vi "LSTM-cell-2 (SubVI).vi"(7 "x":T1, 9 "h":T1, 11 "c":T1) -> (1 "h + 1":T1, 3 "c + 1":T1)   [LabVIEW 2020]
uses:
  <vilib>/Analysis/Matrix/Datatypes/RealMatrix.ctl
  <vilib>/Analysis/7linalg.llb/Real Transpose Matrix.vi
  <vilib>/Analysis/Matrix/Numeric/Conversions/Array To Matrix - RA2.vi
  <vilib>/Analysis/Matrix/Numeric/Add/Add - RM,RM.vi
  <vilib>/Analysis/Matrix/NI_Matrix.lvlib
  <vilib>/Analysis/NI_AALPro.lvlib
panel:
  out "indicator":T1
  in  "bi":T1
  in  "Ui":T1
  in  "Wi":T1
  in  "bc":T1
  in  "Uc":T1
  in  "Wc":T1
  in  "bf":T1
  in  "Uf":T1
  in  "Wf":T1
  in  "bo":T1
  in  "Uo":T1
  in  "Wo":T1
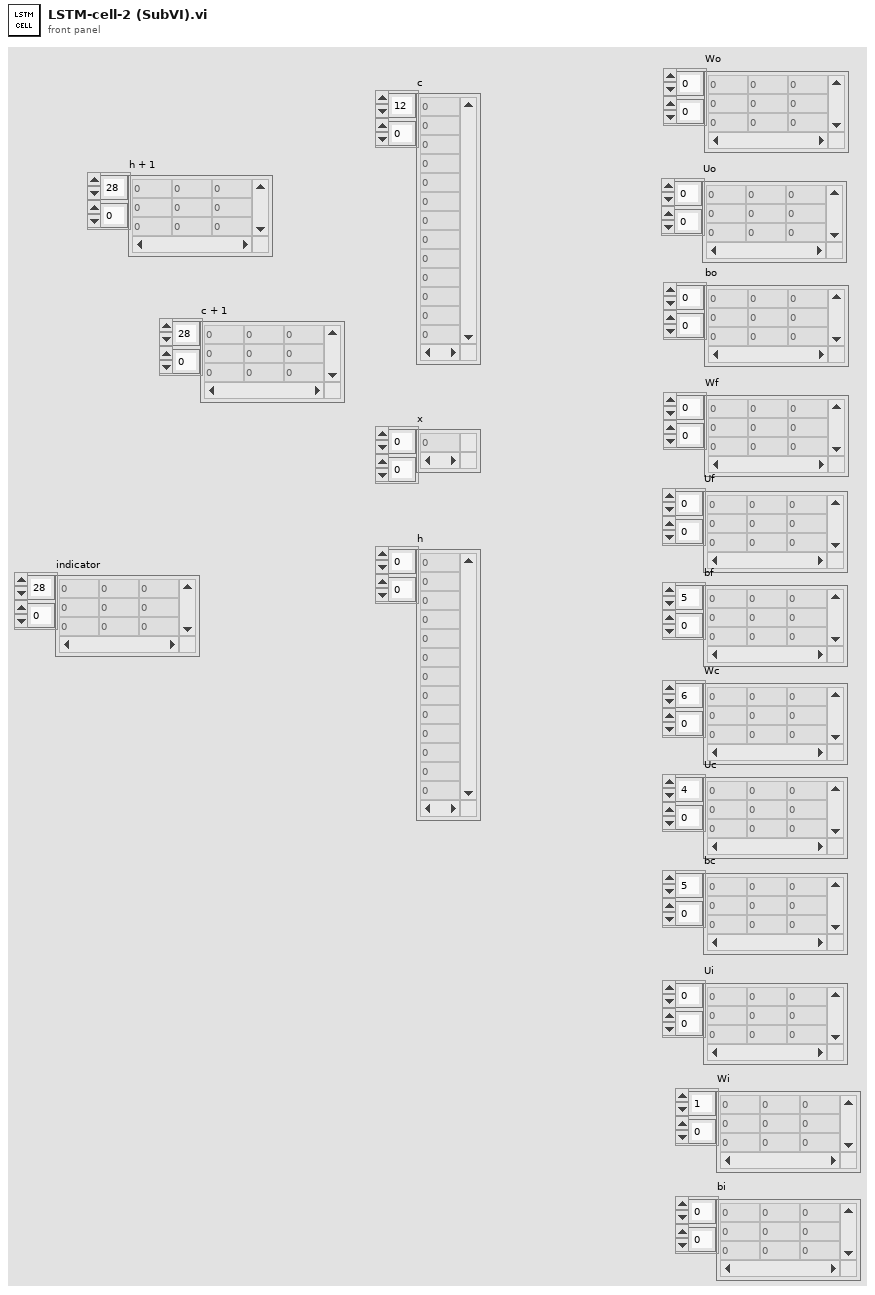
[diagram p1: front panel]
types:
  T1 = typedef "NI_Matrix.lvlib/RealMatrix.ctl" = dbl[][]
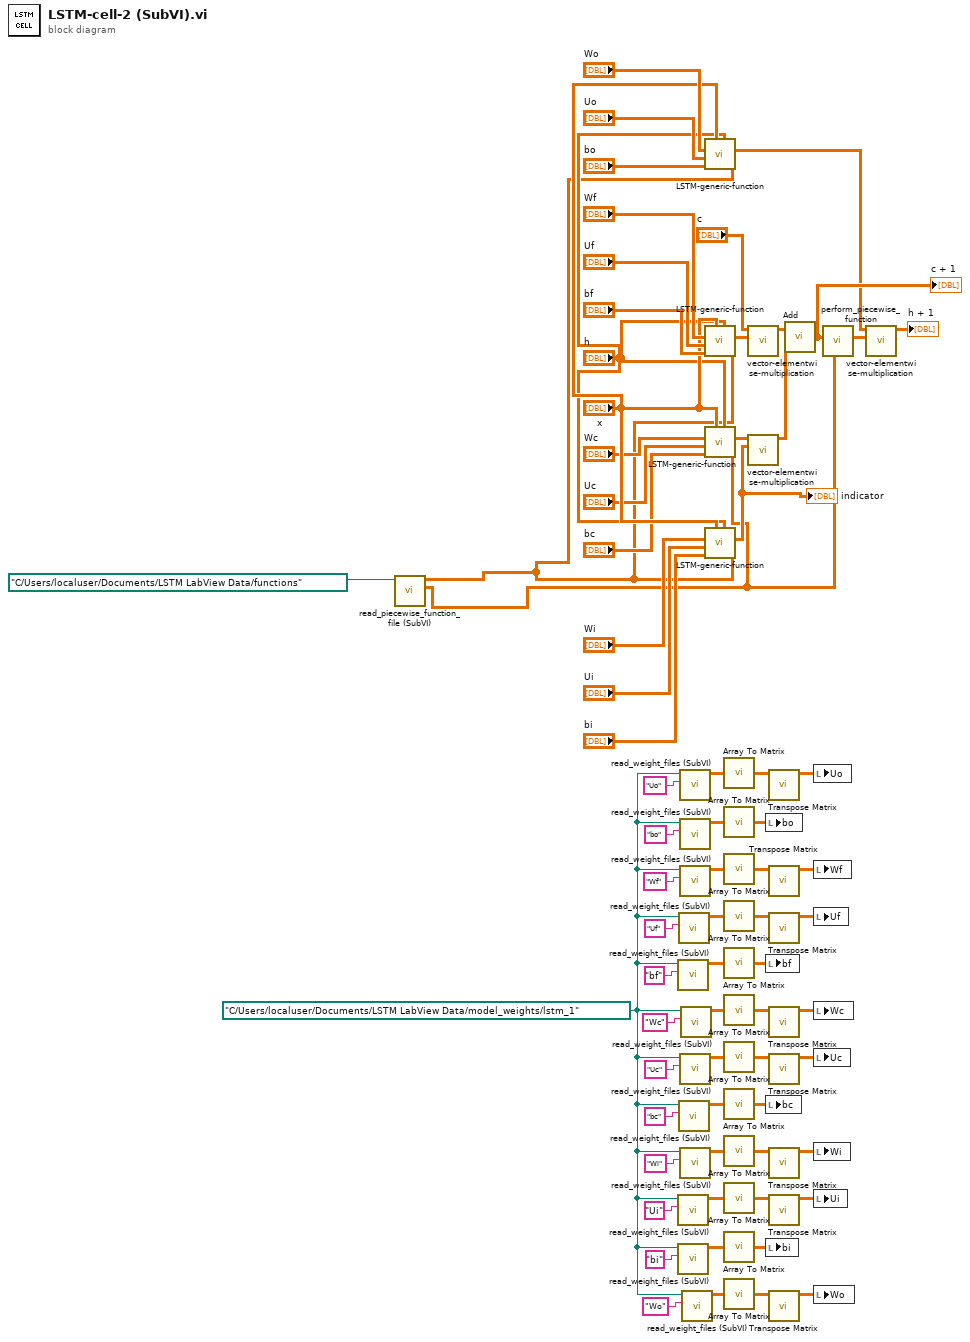
[diagram p0: block diagram]
diagram:
  w46 = path "C:/Users/localuser/Documents/LSTM LabView Data/model_weights/lstm_1" ("cell 1 path")
  n1 = call "read_piecewise_function_file (SubVI).vi"("Path"=path "C:/Users/localuser/Documents/LSTM LabView Data/functions" ("functions path")) -> ("arctan"=w1:dbl[][], "sigmoid"=w2:dbl[][])  [unwired: 9 in]
  n2 = call "read_weight_files (SubVI).vi"("weight file name"="bf" ("String"), "weights path"=w46) -> ("all rows"=w66:dbl[][])  [unwired: 9 in]
  n3 = call "read_weight_files (SubVI).vi"("weight file name"="Ui" ("String"), "weights path"=w46) -> ("all rows"=w60:dbl[][])  [unwired: 9 in]
  n4 = call "read_weight_files (SubVI).vi"("weight file name"="bi" ("String"), "weights path"=w46) -> ("all rows"=w67:dbl[][])  [unwired: 9 in]
  n5 = call "read_weight_files (SubVI).vi"("weight file name"="Uf" ("String"), "weights path"=w46) -> ("all rows"=w62:dbl[][])  [unwired: 9 in]
  n6 = call "read_weight_files (SubVI).vi"("weight file name"="bc" ("String"), "weights path"=w46) -> ("all rows"=w68:dbl[][])  [unwired: 9 in]
  n7 = call "read_weight_files (SubVI).vi"("weight file name"="Uo" ("String"), "weights path"=w46) -> ("all rows"=w65:dbl[][])  [unwired: 9 in]
  n8 = call "read_weight_files (SubVI).vi"("weight file name"="bo" ("String"), "weights path"=w46) -> ("all rows"=w64:dbl[][])  [unwired: 9 in]
  n9 = call "read_weight_files (SubVI).vi"("weight file name"="Wf" ("String"), "weights path"=w46) -> ("all rows"=w63:dbl[][])  [unwired: 9 in]
  n10 = call "read_weight_files (SubVI).vi"("weight file name"="Uc" ("String"), "weights path"=w46) -> ("all rows"=w58:dbl[][])  [unwired: 9 in]
  n11 = call "read_weight_files (SubVI).vi"("weight file name"="Wi" ("String"), "weights path"=w46) -> ("all rows"=w61:dbl[][])  [unwired: 9 in]
  n12 = call "read_weight_files (SubVI).vi"("weight file name"="Wc" ("String"), "weights path"=w46) -> ("all rows"=w59:dbl[][])  [unwired: 9 in]
  n13 = call "read_weight_files (SubVI).vi"("weight file name"="Wo" ("String"), "weights path"=w46) -> ("all rows"=w45:dbl[][])  [unwired: 9 in]
  n14 = call "LSTM-generic-function.vi"("piecewise function"=w2, "h"="h", "x"="x", "b"="bo", "U"="Uo", "W"="Wo") -> ("y"=w21:T1)  [unwired: 5 in]
  n15 = call "LSTM-generic-function.vi"("piecewise function"=w2, "h"="h", "x"="x", "b"="bf", "U"="Uf", "W"="Wf") -> ("y"=w69:T1)  [unwired: 5 in]
  n16 = call "LSTM-generic-function.vi"("piecewise function"=w1, "h"="h", "x"="x", "b"="bc", "U"="Uc", "W"="Wc") -> ("y"=w70:T1)  [unwired: 5 in]
  n17 = call "LSTM-generic-function.vi"("piecewise function"=w2, "h"="h", "x"="x", "b"="bi", "U"="Ui", "W"="Wi") -> ("y"=w4:T1)  [unwired: 5 in]
  "indicator" <- w4
  n18 = call-poly <vilib>:"Array To Matrix.vi"("Real 2D Array"=w65) -> ("Real Matrix"=w42:T1)
  n19 = call-poly <vilib>:"Array To Matrix.vi"("Real 2D Array"=w64) -> ("Real Matrix"=w31:T1)
  n20 = call-poly <vilib>:"Array To Matrix.vi"("Real 2D Array"=w63) -> ("Real Matrix"=w37:T1)
  n21 = call-poly <vilib>:"Array To Matrix.vi"("Real 2D Array"=w62) -> ("Real Matrix"=w40:T1)
  n22 = call-poly <vilib>:"Array To Matrix.vi"("Real 2D Array"=w66) -> ("Real Matrix"=w28:T1)
  n23 = call-poly <vilib>:"Array To Matrix.vi"("Real 2D Array"=w59) -> ("Real Matrix"=w38:T1)
  n24 = call-poly <vilib>:"Array To Matrix.vi"("Real 2D Array"=w58) -> ("Real Matrix"=w41:T1)
  n25 = call-poly <vilib>:"Array To Matrix.vi"("Real 2D Array"=w68) -> ("Real Matrix"=w25:T1)
  n26 = call-poly <vilib>:"Array To Matrix.vi"("Real 2D Array"=w61) -> ("Real Matrix"=w36:T1)
  n27 = call-poly <vilib>:"Array To Matrix.vi"("Real 2D Array"=w60) -> ("Real Matrix"=w39:T1)
  n28 = call-poly <vilib>:"Array To Matrix.vi"("Real 2D Array"=w67) -> ("Real Matrix"=w22:T1)
  n29 = call-poly <vilib>:"Array To Matrix.vi"("Real 2D Array"=w45) -> ("Real Matrix"=w43:T1)
  n30 = call "vector-elementwise-multiplication.vi"("Matrix in"=w69, "Matrix 1"="c") -> ("elementwise product"=w19:T1)  [unwired: 9 in]
  n31 = call "vector-elementwise-multiplication.vi"("Matrix in"=w4, "Matrix 1"=w70) -> ("elementwise product"=w71:T1)  [unwired: 9 in]
  n32 = local write "bo"(w31) -> ()
  n33 = local write "bf"(w28) -> ()
  n34 = local write "bc"(w25) -> ()
  n35 = local write "bi"(w22) -> ()
  n36 = call-poly <vilib>:"Transpose Matrix.vi"("Input Matrix"=w42) -> ("Matrix Transpose"=w32:T1)  [unwired: 9 in, 1 out]
  n37 = call-poly <vilib>:"Transpose Matrix.vi"("Input Matrix"=w37) -> ("Matrix Transpose"=w30:T1)  [unwired: 9 in, 1 out]
  n38 = call-poly <vilib>:"Transpose Matrix.vi"("Input Matrix"=w40) -> ("Matrix Transpose"=w29:T1)  [unwired: 9 in, 1 out]
  n39 = call-poly <vilib>:"Transpose Matrix.vi"("Input Matrix"=w38) -> ("Matrix Transpose"=w27:T1)  [unwired: 9 in, 1 out]
  n40 = call-poly <vilib>:"Transpose Matrix.vi"("Input Matrix"=w41) -> ("Matrix Transpose"=w26:T1)  [unwired: 9 in, 1 out]
  n41 = call-poly <vilib>:"Transpose Matrix.vi"("Input Matrix"=w36) -> ("Matrix Transpose"=w24:T1)  [unwired: 9 in, 1 out]
  n42 = call-poly <vilib>:"Transpose Matrix.vi"("Input Matrix"=w39) -> ("Matrix Transpose"=w23:T1)  [unwired: 9 in, 1 out]
  n43 = call-poly <vilib>:"Transpose Matrix.vi"("Input Matrix"=w43) -> ("Matrix Transpose"=w33:T1)  [unwired: 9 in, 1 out]
  n44 = call-poly <vilib>:"Add.vi"("Real Matrix B"=w71, "Real Matrix A"=w19) -> ("A + B"=w34:T1)
  "c + 1" <- w34
  n45 = local write "Uo"(w32) -> ()
  n46 = local write "Wf"(w30) -> ()
  n47 = local write "Uf"(w29) -> ()
  n48 = local write "Wc"(w27) -> ()
  n49 = local write "Uc"(w26) -> ()
  n50 = local write "Wi"(w24) -> ()
  n51 = local write "Ui"(w23) -> ()
  n52 = local write "Wo"(w33) -> ()
  n53 = call "perform_piecewise_function.vi"("function array"=w1, "x"=w34) -> ("y"=w20:T1)  [unwired: 9 in]
  n54 = call "vector-elementwise-multiplication.vi"("Matrix in"=w20, "Matrix 1"=w21) -> ("elementwise product"=→"h + 1":T1)  [unwired: 9 in]
